vi "Add PV (U16).vi"(6 "initial timestamp":timestamp, 7 "PV name":string, 8 "error in (no error)":errorcluster, 9 "fields":T1, 10 "initial value":u16, 11 "Server in":refnum<class "Server.lvclass">) -> (0 "error out":errorcluster, 2 "value out":u16, 3 "Server out":refnum<class "Server.lvclass">, 4 "timestamp out":timestamp)   [LabVIEW 2020, in "PV Access.lvlib" / "PVA Server.lvlib" / "Server.lvclass"]
uses:
  Server.lvclass
  PV Data/NT Scalar (Numeric)/NT Scalar (Numeric).lvclass
  C:/Users/eyw68381/source/repos/pvaccess-labview/labview/source/PV Data/NT Base/NT Base.lvclass
  Server.lvclass/Server.ctl
  Source/Source.lvclass
  PV Data/PV Data.lvlib
  PV Data/NT Scalar (Numeric)/Create (U16).vi
  PV Data/Value Fields.ctl
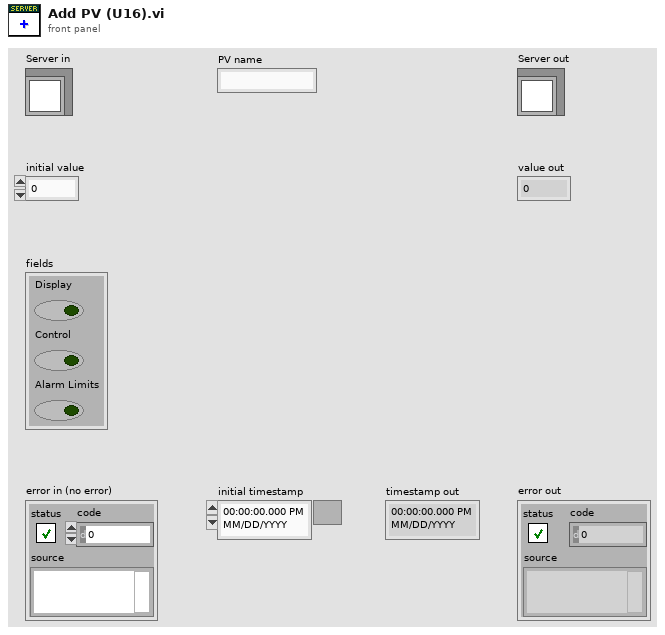
[diagram p1: front panel]
types:
  T1 = typedef "PV Access.lvlib/PV Data.lvlib/Value Fields.ctl" = cluster{"Display":bool, "Control":bool, "Alarm Limits":bool}
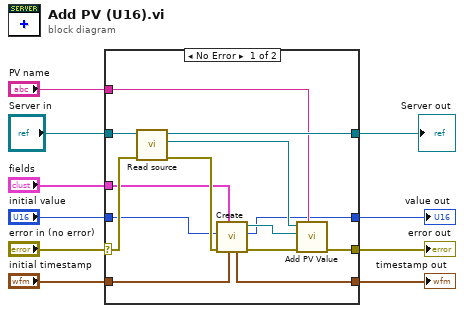
[diagram p0: block diagram]
diagram:
  n1 = case shown="No Error" "error in (no error)" {
    selector: "error in (no error)" -> [w20 w28]
    tunnel: [w19 w28] -> w9
    tunnel: [w23 w27] -> w7
    tunnel: "Server in" -> [w24 w27]
    tunnel: "PV name" -> [w21 _]
    tunnel: "initial value" -> [w15 w26]
    tunnel: [w14 w26] -> w4
    tunnel: "fields" -> [w13 _]
    tunnel: "initial timestamp" -> [w12 w25]
    tunnel: [w11 w25] -> w1
    frame No Error {
      n2 = call "Read source.vi"("error in (no error)"=w20, "Server in"=w24) -> ("error out"=w18:errorcluster, "Source"=w22:refnum<class "Source.lvclass">, "Server out"=w23:refnum<class "Server.lvclass">)  [unwired: 7 in]
      n3 = call-poly "Create.vi"("timestamp in"=w12, "fields"=w13, "error in (no error)"=w18, "value in"=w15) -> ("error out"=w17:errorcluster, "value out"=w14:u16, "NT Scalar (Numeric) out"=w16:refnum<class "NT Scalar (Numeric).lvclass">, "timestamp out"=w11:timestamp)  [unwired: 4 in]
      n4 = call "Add PV Value.vi"("PV name"=w21, "error in"=w17, "NT Base in"=w16, "Source in"=w22) -> ("error out"=w19:errorcluster)  [unwired: 5 in, 2 out]
    }
    frame Error {
    }
  }
  "error out" <- w9
  "Server out" <- w7
  "value out" <- w4
  "timestamp out" <- w1
